vi "GUI_FJ.vi"() -> ()   [LabVIEW 2017]
panel:
  in  "E":bool
  in  "num0 11":bool
  in  "C":bool
  in  "num9":bool
  in  "num8":bool
  in  "num7":bool
  in  "num4 6":bool
  in  "num1 num5":bool
  in  "num6 4":bool
  in  "num3 3":bool
  in  "num2 num2":bool
  in  "num1":bool
  out "Screen":string
  in  "Card Reader":bool
  in  "Terminate Session":bool
  in  "New Transaction":bool
  in  "Fast Cash $50":bool
  in  "Withdrawal":bool
  in  "Deposit":bool
  in  "Balance Inquiry":bool
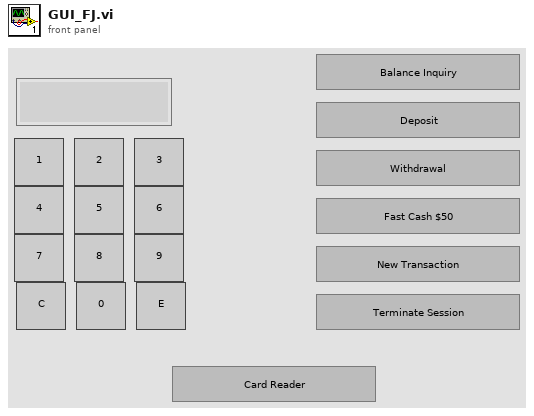
[diagram p1: front panel]
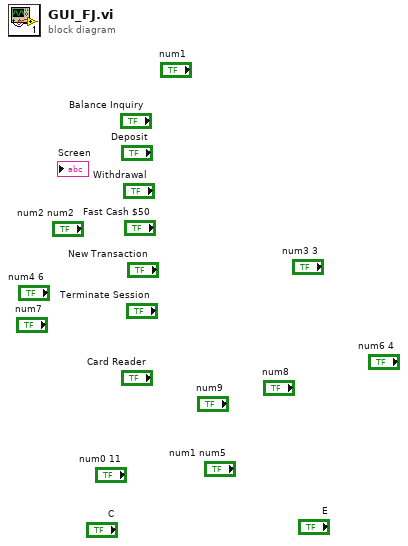
[diagram p0: block diagram]
diagram:
